vi "log_template.vi"(4 "a:ErrorMessage":string="URL=", 6 "a:Success":string, 7 "URL":string="URL=", 8 "StartTime":string, 10 "发送报文":string) -> ()   [LabVIEW 2015]
uses:
  mes/ctl/SenduserRightVerify.ctl
  mes/ctl/SendproCommonInStation.ctl
  mes/ctl/SendproductParaColloctUniversal.ctl
  mes/ctl/SendOutStationCommon.ctl
  mes/ctl/SendEquipStatusCollect.ctl
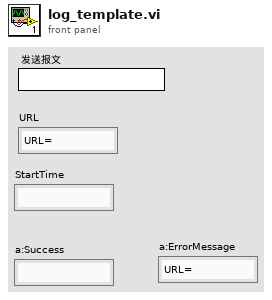
[diagram p1: front panel]
types:
  T1 = enum16{"open", "replace", "create", "open or create", "replace or create", "replace or create with confirmation"}
  T2 = typedef "SenduserRightVerify.ctl" = cluster{"#attributes":cluster{"xmlns:soapenv":string, "xmlns:tem":string, "xmlns:cal":string}, "soapenv:Header":string, "soapenv:Body":cluster{"tem:UserRightVerify":cluster{"tem:model":cluster{"cal:equipNum":string, "cal:passWord":string, "cal:siteCode":string, "cal:userName":string}}}}
  T3 = typedef "SendproCommonInStation.ctl" = cluster{"#attributes":cluster{"xmlns:soapenv":string, "xmlns:tem":string, "xmlns:cal":string}, "soapenv:Header":string, "soapenv:Body":cluster{"tem:ProCommon":cluster{"tem:model":cluster{"cal:equipNum":string, "cal:identification":string, "cal:productType":string, "cal:siteCode":string}}}}
  T4 = typedef "SendproductParaColloctUniversal.ctl" = cluster{"#attributes":cluster{"xmlns:soapenv":string, "xmlns:tem":string, "xmlns:cal":string}, "soapenv:Header":string, "soapenv:Body":cluster{"tem:productParaColloctUniversal":cluster{"tem:vo":cluster{"cal:completeQty":string, "cal:equipNum":string, "cal:identification":string, "cal:productType":string, "cal:qualityStatus":string, "cal:recordDate":string, "cal:siteCode":string, "cal:tagData":cluster{"cal:TagDataVO":cluster{"cal:tagCode":string, "cal:tagValue":string}[]}, "cal:testOrderNum":string, "cal:userName":string}}}}
  T5 = cluster{"cal:tagCode":string, "cal:tagValue":string}[]
  T6 = typedef "SendOutStationCommon.ctl" = cluster{"#attributes":cluster{"xmlns:soapenv":string, "xmlns:tem":string, "xmlns:cal":string}, "soapenv:Header":string, "soapenv:Body":cluster{"tem:outStationService":cluster{"tem:model":cluster{"cal:completeQty":string, "cal:equipNum":string, "cal:identiftyList":cluster{"cal:OutStationVO1":cluster{"cal:identification":string, "cal:qualityStatus":string}[]}, "cal:productType":string, "cal:siteCode":string, "cal:testOrderNum":string}}}}
  T7 = cluster{"cal:identification":string, "cal:qualityStatus":string}[]
  T8 = typedef "SendEquipStatusCollect.ctl" = cluster{"#attributes":cluster{"xmlns:soapenv":string, "xmlns:tem":string, "xmlns:cal":string, "xmlns:arr":string}, "soapenv:Header":string, "soapenv:Body":cluster{"tem:EquipStatusCollect":cluster{"tem:vo":cluster{"cal:equipNum":string, "cal:faultCodes":cluster{"arr:string":string[]}, "cal:recordDate":string, "cal:remarks":string, "cal:siteCode":string, "cal:statusCode":string, "cal:userName":string}}}}
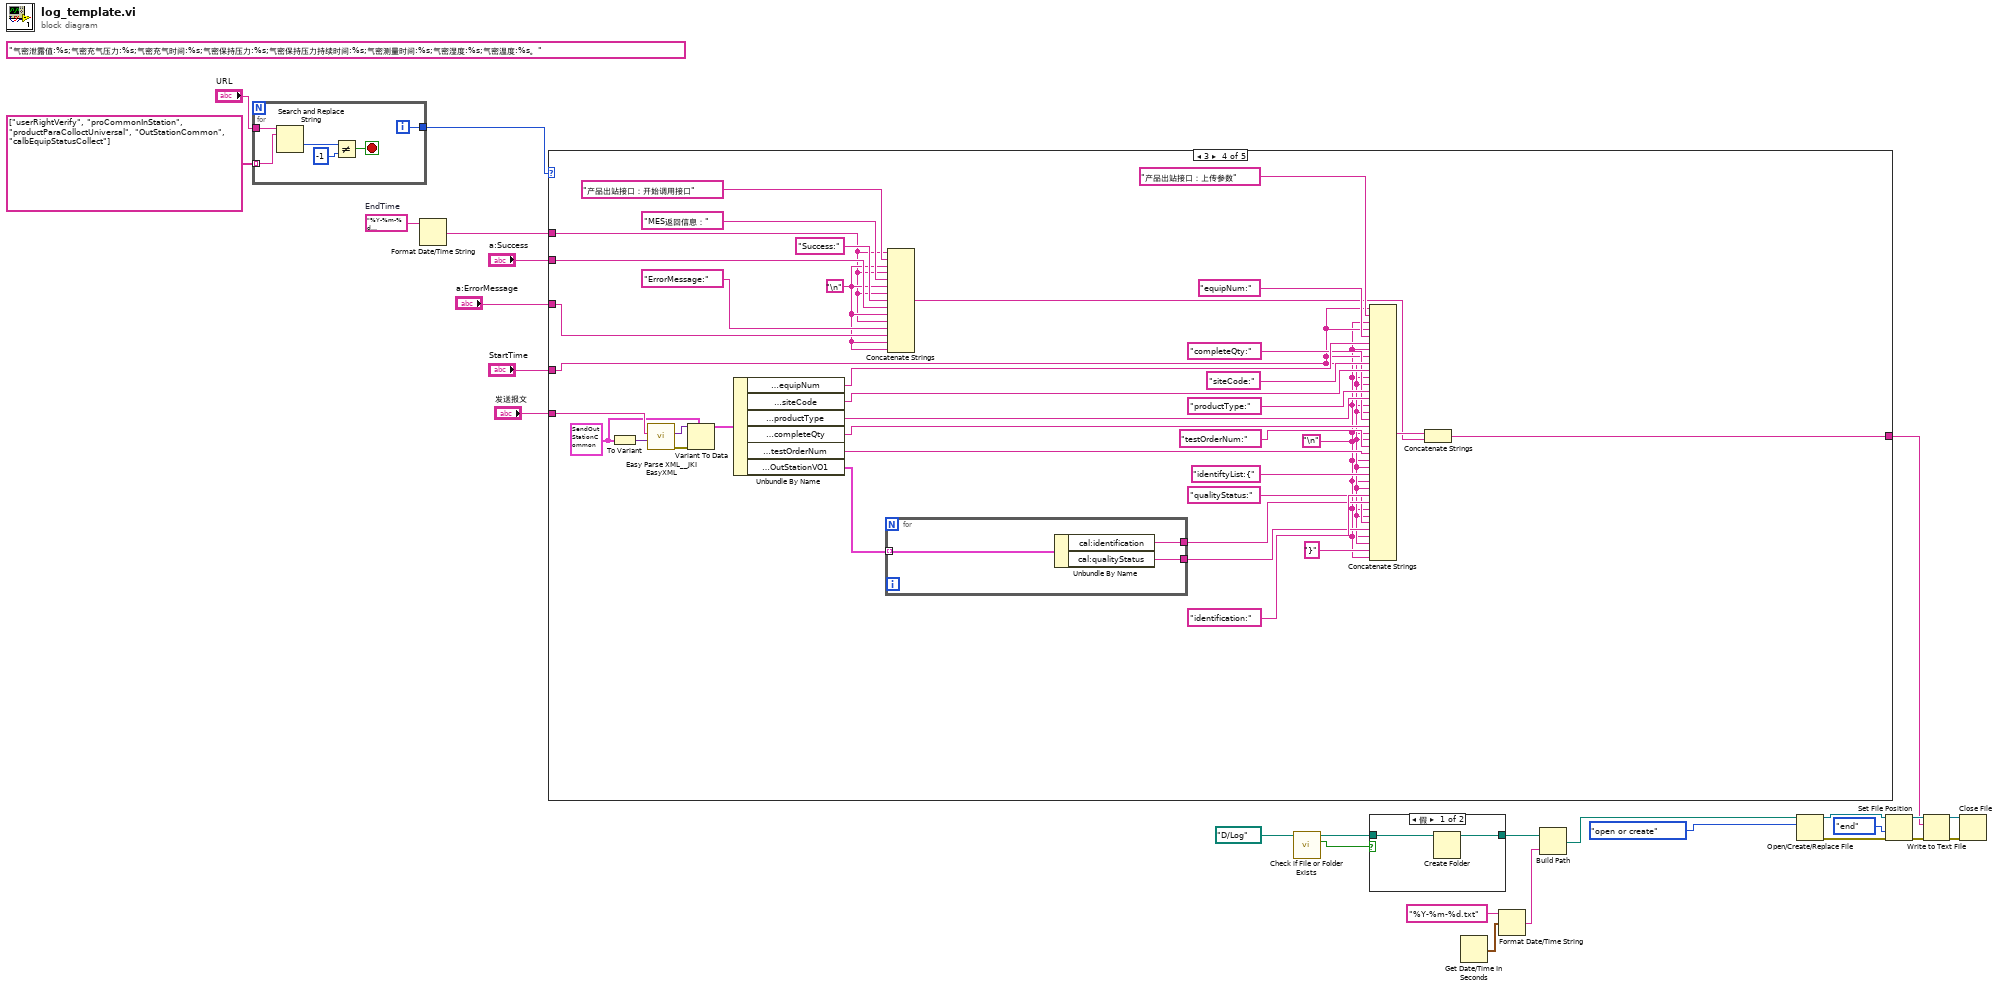
[diagram p0: block diagram]
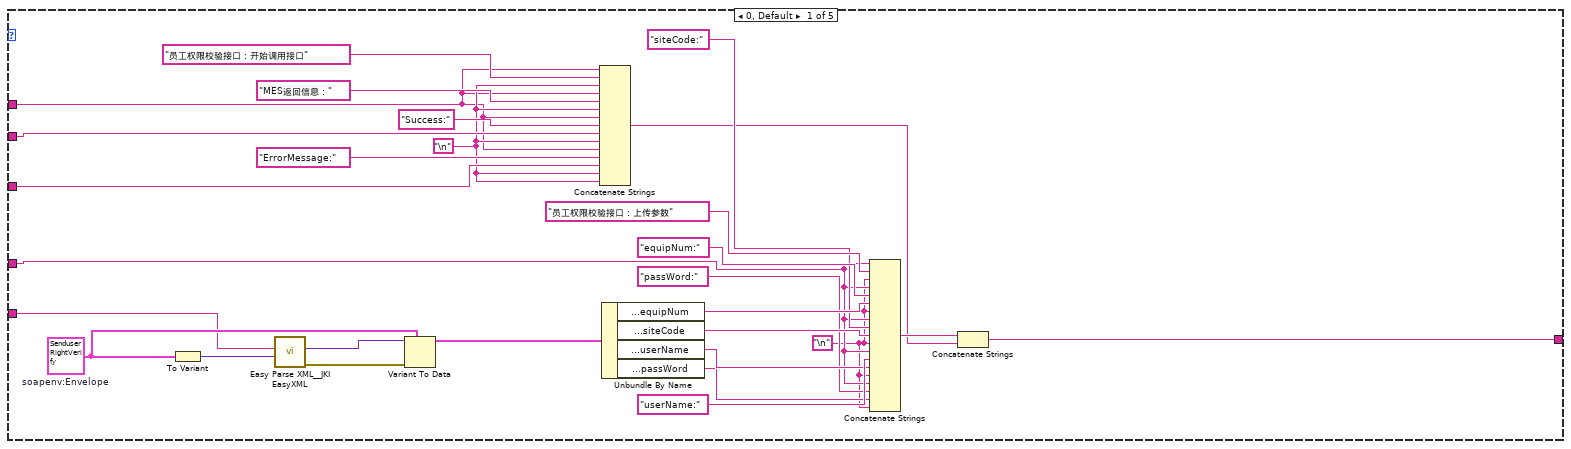
[diagram p2: hidden frame]
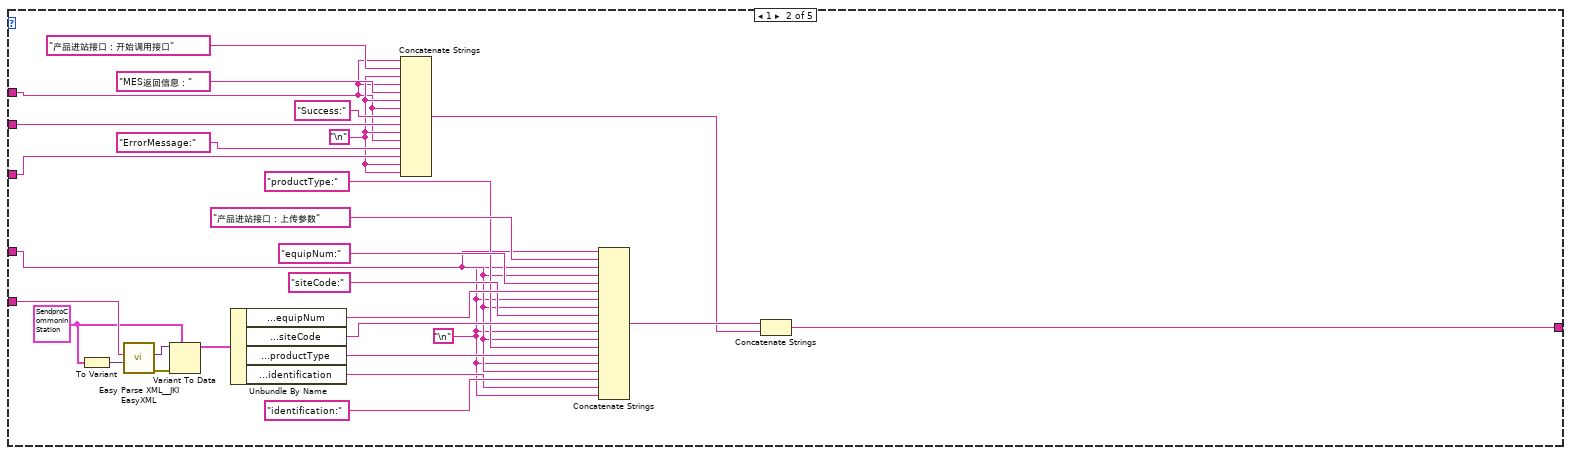
[diagram p3: hidden frame]
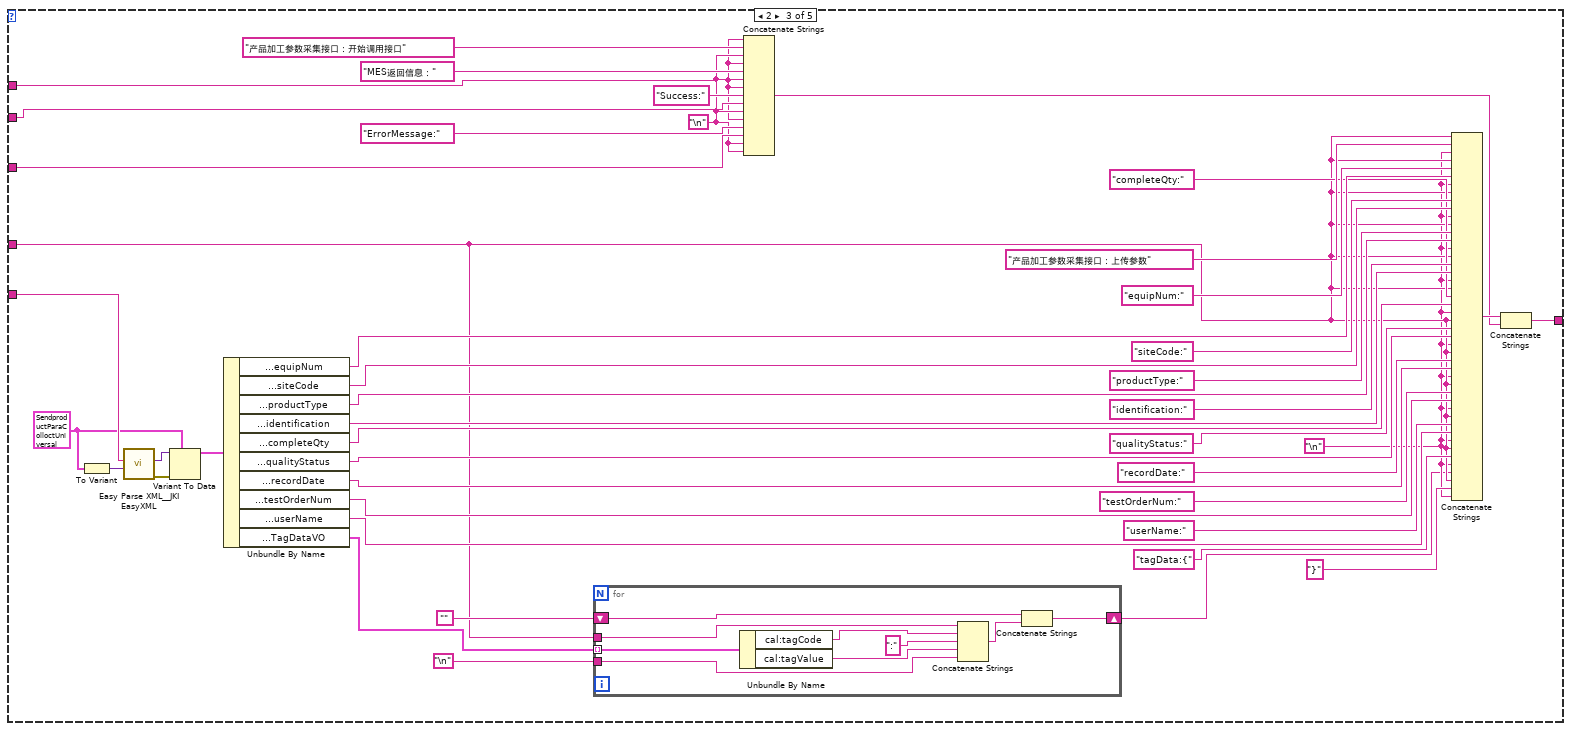
[diagram p4: hidden frame]
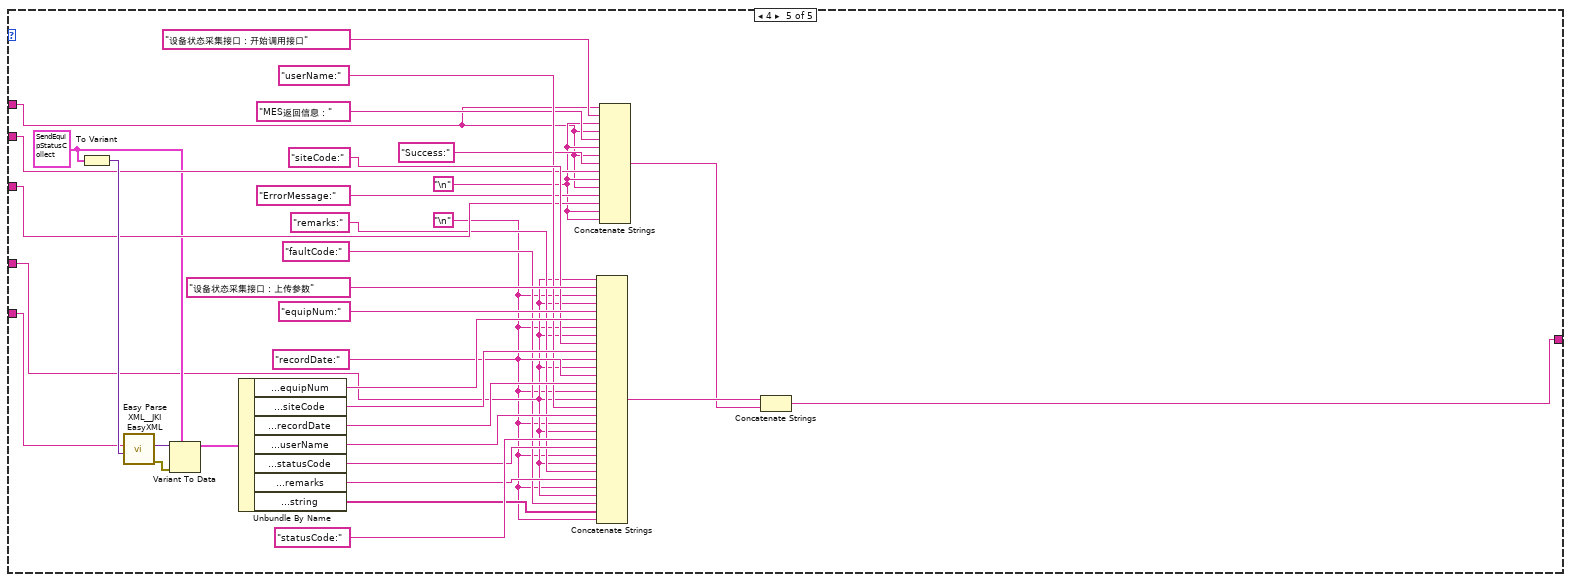
[diagram p5: hidden frame]
diagram:
  w14 = "%Y-%m-%d %H:%M:%S%3u-->"  # EndTime
  (unwired) "气密泄露值:%s;气密充气压力:%s;气密充气时间:%s;气密保持压力:%s;气密保持压力持续时间:%s;气密测量时间:%s;气密湿度:%s;气密温度:%s。" ("value")
  n1 = for {
    tunnel: string[] ["userRightVerify", "proCommonInStation", "productParaColloctUniversal", "OutStationCommon", "calbEquipStatusCollect"] ("字符串数组") -> [w28] mode=indexing
    tunnel: "URL" -> [w32]
    tunnel: [w27] -> w18
    i -> [w27]
    stop <- w29 stop-if-true
    n2 = Search and Replace String(input string=w32, search string=w28) -> (offset past replacement=w30:i32)  [unwired: 6 in, 3 out]
    n3 = Not Equal?(x=w30, y=-1) -> (x != y?=w29:bool)
  }
  n4 = Format Date/Time String(time format string (%c)=w14) -> (date/time string=w13:string)  [unwired: 2 in]
  n5 = case shown="3" w18 {
    tunnel: "发送报文" -> [w56 w85 w129 w175 w212]
    tunnel: "StartTime" -> [w47 w76 w92 w144 w185]
    tunnel: w13 -> [w36 w65 w111 w157 w194]
    tunnel: "a:Success" -> [w40 w69 w115 w161 w198]
    tunnel: "a:ErrorMessage" -> [w38 w67 w113 w159 w196]
    tunnel: [w33 w62 w108 w154 w191] -> w3
    frame 0, Default {
      w37 = "\n"
      w57 = T2 {"#attributes"={"xmlns:soapenv"="http://schemas.xmlsoap.org/soap/envelope/", "xmlns:tem"="http://tempuri.org/", "xmlns:cal"="http://schemas.datacontract.org/2004/07/CalbUserRightVerifyService"}, "soapenv:Header"="", "soapenv:Body"={"tem:UserRightVerify"={"tem:model"={"cal:equipNum"="", "cal:passWord"="", "cal:siteCode"="", "cal:userName"=""}}}}  # soapenv:Envelope
      w44 = "\n"
      n6 = To Variant(anything=w57) -> (Variant=w59:variant)
      n7 = call <vilib>:"Easy Parse XML__JKI EasyXML.vi"("LabVIEW Data (Type)"=w59, "XML String"=w56) -> ("error out"=w55:errorcluster, "LabVIEW Data"=w58:variant)  [unwired: 8 in]
      n8 = Variant To Data(error in=w55, type=w57, Variant=w58) -> (data=w54:T2)  [unwired: 1 out]
      n9 = Concatenate Strings(w36, "员工权限校验接口：开始调用接口", w37, w36, "MES返回信息：", w37, w36, "Success:", w40, w37, w36, "ErrorMessage:", w38, w37, w37) -> (w34:string)
      n10 = Unbundle By Name(w54) -> ("soapenv:Body.tem:UserRightVerify.tem:model.cal:equipNum"=w52:string, "soapenv:Body.tem:UserRightVerify.tem:model.cal:siteCode"=w51:string, "soapenv:Body.tem:UserRightVerify.tem:model.cal:userName"=w48:string, "soapenv:Body.tem:UserRightVerify.tem:model.cal:passWord"=w45:string)
      n11 = Concatenate Strings(w47, "员工权限校验接口：上传参数", w44, w47, "equipNum:", w52, w44, w47, "siteCode:", w51, w44, w47, "userName:", w48, w44, w47, "passWord:", w45, w44) -> (w35:string)
      n12 = Concatenate Strings(w35, w34) -> (w33:string)
    }
    frame 1 {
      w61 = T3 {"#attributes"={"xmlns:soapenv"="http://schemas.xmlsoap.org/soap/envelope/", "xmlns:tem"="http://tempuri.org/", "xmlns:cal"="http://schemas.datacontract.org/2004/07/CalbProCommonInStationService"}, "soapenv:Header"="", "soapenv:Body"={"tem:ProCommon"={"tem:model"={"cal:equipNum"="", "cal:identification"="", "cal:productType"="", "cal:siteCode"=""}}}} ("soapenv:Envelope")
      w66 = "\n"
      w73 = "\n"
      n13 = To Variant(anything=w61) -> (Variant=w87:variant)
      n14 = call <vilib>:"Easy Parse XML__JKI EasyXML.vi"("LabVIEW Data (Type)"=w87, "XML String"=w85) -> ("error out"=w84:errorcluster, "LabVIEW Data"=w86:variant)  [unwired: 8 in]
      n15 = Variant To Data(error in=w84, type=w61, Variant=w86) -> (data=w83:T3)  [unwired: 1 out]
      n16 = Unbundle By Name(w83) -> ("soapenv:Body.tem:ProCommon.tem:model.cal:equipNum"=w81:string, "soapenv:Body.tem:ProCommon.tem:model.cal:siteCode"=w80:string, "soapenv:Body.tem:ProCommon.tem:model.cal:productType"=w77:string, "soapenv:Body.tem:ProCommon.tem:model.cal:identification"=w74:string)
      n17 = Concatenate Strings(w65, "产品进站接口：开始调用接口", w66, w65, "MES返回信息：", w66, w65, "Success:", w69, w66, w65, "ErrorMessage:", w67, w66, w66) -> (w63:string)
      n18 = Concatenate Strings(w76, "产品进站接口：上传参数", w73, w76, "equipNum:", w81, w73, w76, "siteCode:", w80, w73, w76, "productType:", w77, w73, w76, "identification:", w74, w73) -> (w64:string)
      n19 = Concatenate Strings(w64, w63) -> (w62:string)
    }
    frame 2 {
      w107 = T4 {"#attributes"={"xmlns:soapenv"="http://schemas.xmlsoap.org/soap/envelope/", "xmlns:tem"="http://tempuri.org/", "xmlns:cal"="http://schemas.datacontract.org/2004/07/CalbProductParaColloctUniversalService"}, "soapenv:Header"="", "soapenv:Body"={"tem:productParaColloctUniversal"={"tem:vo"={"cal:completeQty"="", "cal:equipNum"="", "cal:identification"="", "cal:productType"="", "cal:qualityStatus"="", "cal:recordDate"="", "cal:siteCode"="", "cal:tagData"={"cal:TagDataVO"=[]}, "cal:testOrderNum"="", "cal:userName"=""}}}} ("soapenv:Envelope")
      w112 = "\n"
      w90 = "\n"
      n20 = To Variant(anything=w107) -> (Variant=w131:variant)
      n21 = call <vilib>:"Easy Parse XML__JKI EasyXML.vi"("LabVIEW Data (Type)"=w131, "XML String"=w129) -> ("error out"=w128:errorcluster, "LabVIEW Data"=w130:variant)  [unwired: 8 in]
      n22 = Variant To Data(error in=w128, type=w107, Variant=w130) -> (data=w127:T4)  [unwired: 1 out]
      n23 = Unbundle By Name(w127) -> ("soapenv:Body.tem:productParaColloctUniversal.tem:vo.cal:equipNum"=w125:string, "soapenv:Body.tem:productParaColloctUniversal.tem:vo.cal:siteCode"=w124:string, "soapenv:Body.tem:productParaColloctUniversal.tem:vo.cal:productType"=w121:string, "soapenv:Body.tem:productParaColloctUniversal.tem:vo.cal:identification"=w119:string, "soapenv:Body.tem:productParaColloctUniversal.tem:vo.cal:completeQty"=w105:string, "soapenv:Body.tem:productParaColloctUniversal.tem:vo.cal:qualityStatus"=w103:string, "soapenv:Body.tem:productParaColloctUniversal.tem:vo.cal:recordDate"=w101:string, "soapenv:Body.tem:productParaColloctUniversal.tem:vo.cal:testOrderNum"=w99:string, "soapenv:Body.tem:productParaColloctUniversal.tem:vo.cal:userName"=w97:string, "soapenv:Body.tem:productParaColloctUniversal.tem:vo.cal:tagData.cal:TagDataVO"=w93:T5)
      n24 = for {
        tunnel: w93 -> [w141] mode=indexing
        tunnel: w92 -> [w137]
        tunnel: "\n" -> [w136]
        shift-right: [w133] -> w89
        shift-left: "" -> [w135]
        n25 = Unbundle By Name(w141) -> ("cal:tagCode"=w140:string, "cal:tagValue"=w138:string)
        n26 = Concatenate Strings(w137, w140, ":" ("字符串"), w138, w136) -> (w134:string)
        n27 = Concatenate Strings(w135, w134) -> (w133:string)
      }
      n28 = Concatenate Strings(w111, "产品加工参数采集接口：开始调用接口", w112, w111, "MES返回信息：", w112, w111, "Success:", w115, w112, w111, "ErrorMessage:", w113, w112, w112) -> (w109:string)
      n29 = Concatenate Strings(w92, "产品加工参数采集接口：上传参数", w90, w92, "equipNum:", w125, w90, w92, "siteCode:", w124, w90, w92, "productType:", w121, w90, w92, "identification:", w119, w90, w92, "completeQty:", w105, w90, w92, "qualityStatus:", w103, w90, w92, "recordDate:", w101, w90, w92, "testOrderNum:", w99, w90, w92, "userName:", w97, w90, w92, "tagData:{", w90, w89, w92, "}", w90) -> (w110:string)
      n30 = Concatenate Strings(w110, w109) -> (w108:string)
    }
    frame 3 {
      w153 = T6 {"#attributes"={"xmlns:soapenv"="http://schemas.xmlsoap.org/soap/envelope/", "xmlns:tem"="http://tempuri.org/", "xmlns:cal"="http://schemas.datacontract.org/2004/07/CalbOutStationCommonService"}, "soapenv:Header"="", "soapenv:Body"={"tem:outStationService"={"tem:model"={"cal:completeQty"="", "cal:equipNum"="", "cal:identiftyList"={"cal:OutStationVO1"=[]}, "cal:productType"="", "cal:siteCode"="", "cal:testOrderNum"=""}}}} ("soapenv:Envelope")
      w158 = "\n"
      w142 = "\n"
      n31 = To Variant(anything=w153) -> (Variant=w177:variant)
      n32 = call <vilib>:"Easy Parse XML__JKI EasyXML.vi"("LabVIEW Data (Type)"=w177, "XML String"=w175) -> ("error out"=w174:errorcluster, "LabVIEW Data"=w176:variant)  [unwired: 8 in]
      n33 = Variant To Data(error in=w174, type=w153, Variant=w176) -> (data=w173:T6)  [unwired: 1 out]
      n34 = Unbundle By Name(w173) -> ("soapenv:Body.tem:outStationService.tem:model.cal:equipNum"=w171:string, "soapenv:Body.tem:outStationService.tem:model.cal:siteCode"=w170:string, "soapenv:Body.tem:outStationService.tem:model.cal:productType"=w167:string, "soapenv:Body.tem:outStationService.tem:model.cal:completeQty"=w165:string, "soapenv:Body.tem:outStationService.tem:model.cal:testOrderNum"=w151:string, "soapenv:Body.tem:outStationService.tem:model.cal:identiftyList.cal:OutStationVO1"=w149:T7)
      n35 = for {
        tunnel: w149 -> [w181] mode=indexing
        tunnel: [w180] -> w147
        tunnel: [w179] -> w145
        n36 = Unbundle By Name(w181) -> ("cal:identification"=w180:string, "cal:qualityStatus"=w179:string)
      }
      n37 = Concatenate Strings(w157, "产品出站接口：开始调用接口", w158, w157, "MES返回信息：", w158, w157, "Success:", w161, w158, w157, "ErrorMessage:", w159, w158, w158) -> (w155:string)
      n38 = Concatenate Strings(w144, "产品出站接口：上传参数", w142, w144, "equipNum:", w171, w142, w144, "siteCode:", w170, w142, w144, "productType:", w167, w142, w144, "completeQty:", w165, w142, w144, "testOrderNum:", w151, w142, w144, "identiftyList:{", w142, w144, "identification:", w147, w142, w144, "qualityStatus:", w145, w142, w144, "}" ("字符串"), w142) -> (w156:string)
      n39 = Concatenate Strings(w156, w155) -> (w154:string)
    }
    frame 4 {
      w187 = T8 {"#attributes"={"xmlns:soapenv"="http://schemas.xmlsoap.org/soap/envelope/", "xmlns:tem"="http://tempuri.org/", "xmlns:cal"="http://schemas.datacontract.org/2004/07/CalbEquipStatusCollectService", "xmlns:arr"="http://schemas.microsoft.com/2003/10/Serialization/Arrays"}, "soapenv:Header"="", "soapenv:Body"={"tem:EquipStatusCollect"={"tem:vo"={"cal:equipNum"="", "cal:faultCodes"={"arr:string"=[]}, "cal:recordDate"="", "cal:remarks"="", "cal:siteCode"="", "cal:statusCode"="", "cal:userName"=""}}}} ("soapenv:Envelope")
      w195 = "\n"
      w182 = "\n"
      n40 = To Variant(anything=w187) -> (Variant=w214:variant)
      n41 = call <vilib>:"Easy Parse XML__JKI EasyXML.vi"("LabVIEW Data (Type)"=w214, "XML String"=w212) -> ("error out"=w211:errorcluster, "LabVIEW Data"=w213:variant)  [unwired: 8 in]
      n42 = Variant To Data(error in=w211, type=w187, Variant=w213) -> (data=w210:T8)  [unwired: 1 out]
      n43 = Unbundle By Name(w210) -> ("soapenv:Body.tem:EquipStatusCollect.tem:vo.cal:equipNum"=w208:string, "soapenv:Body.tem:EquipStatusCollect.tem:vo.cal:siteCode"=w207:string, "soapenv:Body.tem:EquipStatusCollect.tem:vo.cal:recordDate"=w204:string, "soapenv:Body.tem:EquipStatusCollect.tem:vo.cal:userName"=w202:string, "soapenv:Body.tem:EquipStatusCollect.tem:vo.cal:statusCode"=w189:string, "soapenv:Body.tem:EquipStatusCollect.tem:vo.cal:remarks"=w186:string, "soapenv:Body.tem:EquipStatusCollect.tem:vo.cal:faultCodes.arr:string"=w183:string[])
      n44 = Concatenate Strings(w185, "设备状态采集接口：上传参数", w182, w185, "equipNum:", w208, w182, w185, "siteCode:", w207, w182, w185, "recordDate:", w204, w182, w185, "userName:", w202, w182, w185, "statusCode:", w189, w182, w185, "remarks:", w186, w182, w185, "faultCode:", w183, w182) -> (w193:string)
      n45 = Concatenate Strings(w194, "设备状态采集接口：开始调用接口", w195, w194, "MES返回信息：", w195, w194, "Success:", w198, w195, w194, "ErrorMessage:", w196, w195, w195) -> (w192:string)
      n46 = Concatenate Strings(w193, w192) -> (w191:string)
    }
  }
  n47 = call <vilib>:"Check if File or Folder Exists.vi"("path"=path "D:/Log" ("路径")) -> ("file or folder exists?"=w24:bool, "dup path"=w25:path)  [unwired: 8 in, 1 out]
  n48 = case shown="假" w24 {
    tunnel: w25 -> [w217 w218]
    tunnel: [w216 w218] -> w22
    frame False {
      n49 = Create Folder(path (use dialog)=w217) -> (created path=w216:path)  [unwired: 2 in, 2 out]
    }
    frame True {
    }
  }
  n50 = Get Date/Time In Seconds() -> (seconds since 1Jan1904=w20:timestamp)
  n51 = Format Date/Time String(time format string (%c)="%Y-%m-%d.txt" ("时间格式字符串(%c)"), seconds (now)=w20) -> (date/time string=w19:string)  [unwired: 1 in]
  n52 = Build Path(base path=w22, name or relative path=w19) -> (appended path=w26:path)
  n53 = Open/Create/Replace File(file path (use dialog)=w26, operation (0:open)=T1."open or create" ("操作(0:open)")) -> (refnum out=w7:refnum<file>, error out=w8:errorcluster)  [unwired: 4 in, 1 out]
  n54 = Set File Position(refnum=w7, from (0:start)=enum16{"start", "end", "current"}."end" ("自（0:起始）"), error in=w8) -> (refnum out=w9:refnum<file>, error out=w10:errorcluster)  [unwired: 1 in]
  n55 = Write to Text File(file (use dialog)=w9, text=w3, error in=w10) -> (refnum out=w6:refnum<file>, error out=w5:errorcluster)  [unwired: 1 in, 1 out]
  n56 = Close File(refnum=w6, error in=w5) -> ()  [unwired: 2 out]
